vi "clock.vi"() -> ()   [LabVIEW 2019]
uses:
  <vilib>/rvi/Emulation/niFpgaGetClockAttributes.vi
  <vilib>/rvi/Emulation/niFpgaSctlEmulationGetInTimedLoop.vi
  <vilib>/rvi/Emulation/niFpgaEmulationReportErrorSimple.vi
  <vilib>/rvi/eio/common/nirviEmuTemplateMethod_errors.vi
  <vilib>/rvi/Emulation/niFpgaCriticalErrorInLSC.vi
  <vilib>/eio/EIONode/EIONode.xnode
panel:
  in  "stop":bool
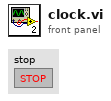
[diagram p1: front panel]
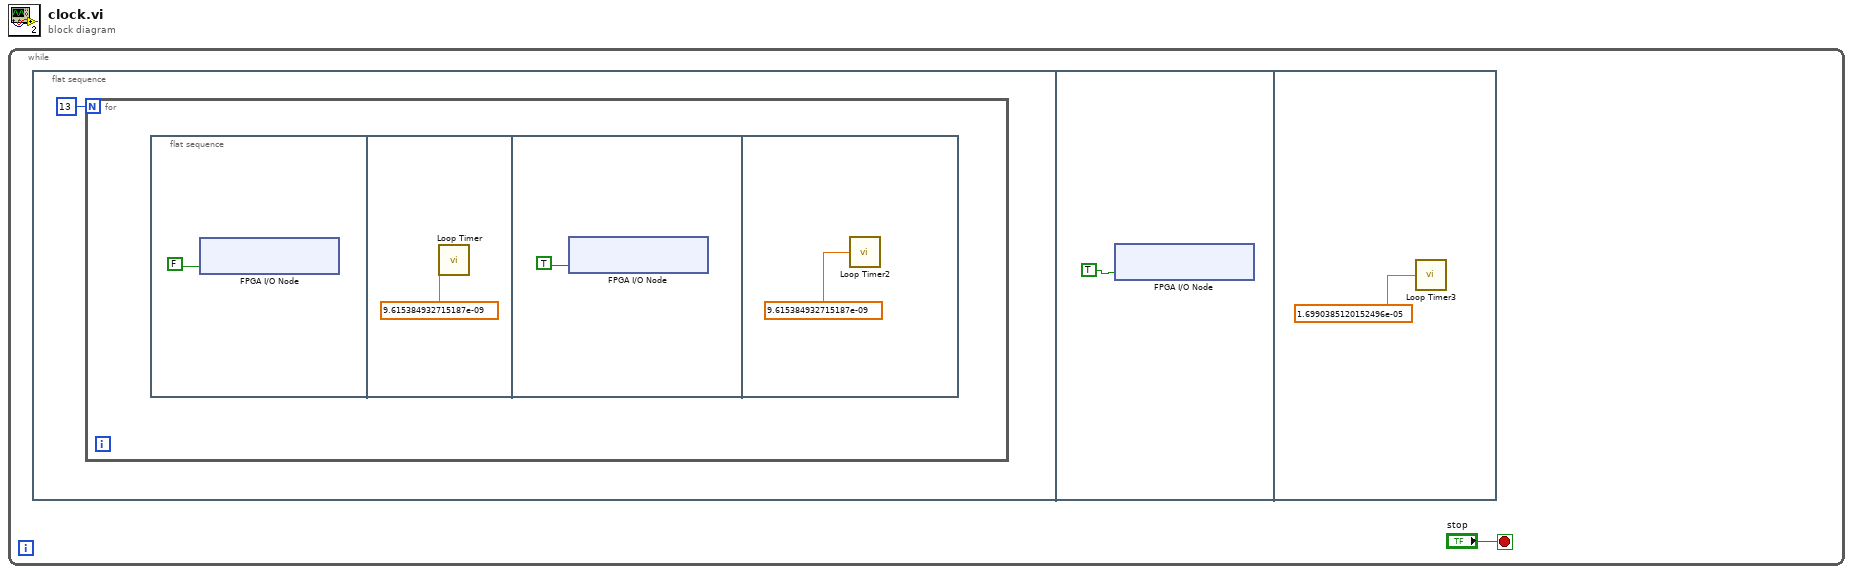
[diagram p0: block diagram]
diagram:
  n1 = while {
    stop <- "stop" stop-if-true
    n2 = flat-sequence {
      frame #0 {
        n3 = for {
          N: 13 -> [_]
          n4 = flat-sequence {
            frame #0 {
              n5 = xnode "FPGA I/O Node"("ConnectorB/DIO7"=FALSE) -> ()  [unwired: 1 in, 1 out]
            }
            frame #1 {
              n6 = call "Loop Timer"("Count(Ticks)"=sgl 9.615385e-09) -> ()  [unwired: 1 out]
            }
            frame #2 {
              n7 = xnode "FPGA I/O Node"("ConnectorB/DIO7"=TRUE) -> ()  [unwired: 1 in, 1 out]
            }
            frame #3 {
              n8 = call "Loop Timer2"("Count(Ticks)"=sgl 9.615385e-09) -> ()  [unwired: 1 out]
            }
          }
        }
      }
      frame #1 {
        n9 = xnode "FPGA I/O Node"("ConnectorB/DIO7"=TRUE) -> ()  [unwired: 1 in, 1 out]
      }
      frame #2 {
        n10 = call "Loop Timer3"("Count(Ticks)"=sgl 1.6990385e-05) -> ()  [unwired: 1 out]
      }
    }
  }
